vi "Get Device Channel Info.vi"(8 "error in":errorcluster, 10 "Channel Data in":T1 {"Device Chan Total" max=32 step=1; "Thermocouple"."Temperature Units" items=["Celcius", "Fahrenheit", "Kelvin", "Rankine", "Volts"]; "Thermocouple"."Thermocouple Type" items=["J", "K", "T", "E", "N", "B", "R", "S", "Raw Voltage"]}, 11 "Custom Device Ref in":T5 format="%.0x") -> (0 "error out":errorcluster, 2 "Channel Data out":T1 {"Device Chan Total" max=32 step=1; "Thermocouple"."Temperature Units" items=["Celcius", "Fahrenheit", "Kelvin", "Rankine", "Volts"]; "Thermocouple"."Thermocouple Type" items=["J", "K", "T", "E", "N", "B", "R", "S", "Raw Voltage"]}, 3 "Device Configuration Data":T4 {"Current Section Ref" format="%.0x"; "simTC Section Refs" format="%.0x"; "Voltage Section Ref" format="%.0x"; "Custom Device Ref" format="%.0x"})   [LabVIEW 2011, in "Simulated Thermocouple Custom Device.lvlib"]
uses:
  Simulated Thermocouple Custom Device.lvlib
  <vilib>/NI Veristand/Custom Device API/Custom Device Item Ref.ctl
  Device Config data.ctl
  New Channel Data.ctl
  TC Selector.ctl
  TC Unit Selector.ctl
  Device Settings.ctl
  TC Section Config Data.ctl
  <vilib>/NI Veristand/Custom Device API/Get Item Property (Variant).vi
  simTC Global GUIDs.vi
  <vilib>/NI Veristand/Custom Device Tools/Custom Device Utility Library/NI VeriStand - Search for All Items by GUID.vi
  <vilib>/NI Veristand/Custom Device Tools/Custom Device Utility Library/NI VeriStand - Search for Item by GUID.vi
  <vilib>/NI Veristand/Custom Device API/Get Item Property (String).vi
  <vilib>/NI Veristand/Custom Device Tools/Custom Device Utility Library/Custom Device Utility Library.lvlib
  <vilib>/NI Veristand/Custom Device API/Custom Device API.lvlib
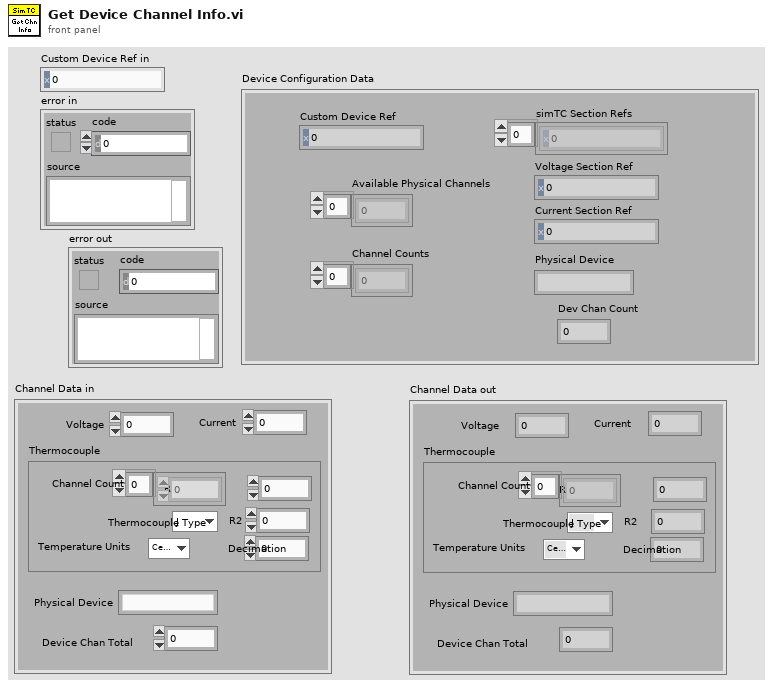
[diagram p1: front panel]
types:
  T1 = typedef "Simulated Thermocouple Custom Device.lvlib/New Channel Data.ctl" = cluster{"Voltage":u32, "Current":u32, "Thermocouple":cluster{"R1":dbl, "R2":dbl, "Decimation":u32, "Thermocouple Type":T2, "Temperature Units":T3, "Channel Count":u32[]}, "Physical Device":string, "Device Chan Total":u32}
  T2 = typedef "Simulated Thermocouple Custom Device.lvlib/TC Selector.ctl" = u16
  T3 = typedef "Simulated Thermocouple Custom Device.lvlib/TC Unit Selector.ctl" = u16
  T4 = typedef "Simulated Thermocouple Custom Device.lvlib/Device Config data.ctl" = cluster{"Custom Device Ref":T5, "Voltage Section Ref":T5, "simTC Section Refs":T5[], "Current Section Ref":T5, "Physical Device":string, "Available Physical Channels":i32[], "Channel Counts":u32[], "Dev Chan Count":u32}
  T5 = typedef "Custom Device API.lvlib/Custom Device Item Ref.ctl" = u64
  T6 = typedef "Simulated Thermocouple Custom Device.lvlib/Device Settings.ctl" = cluster{"High Side Resistance (Ohms)":dbl, "Low Side Resistance (Ohms)":dbl, "Temperature Units":T3, "Update Rate":dbl, "Physical Device Name":string, "Device Channel Count":u32}
  T7 = typedef "Simulated Thermocouple Custom Device.lvlib/TC Section Config Data.ctl" = cluster{"Temperature Units":T3, "Thermocouple Type":T2}
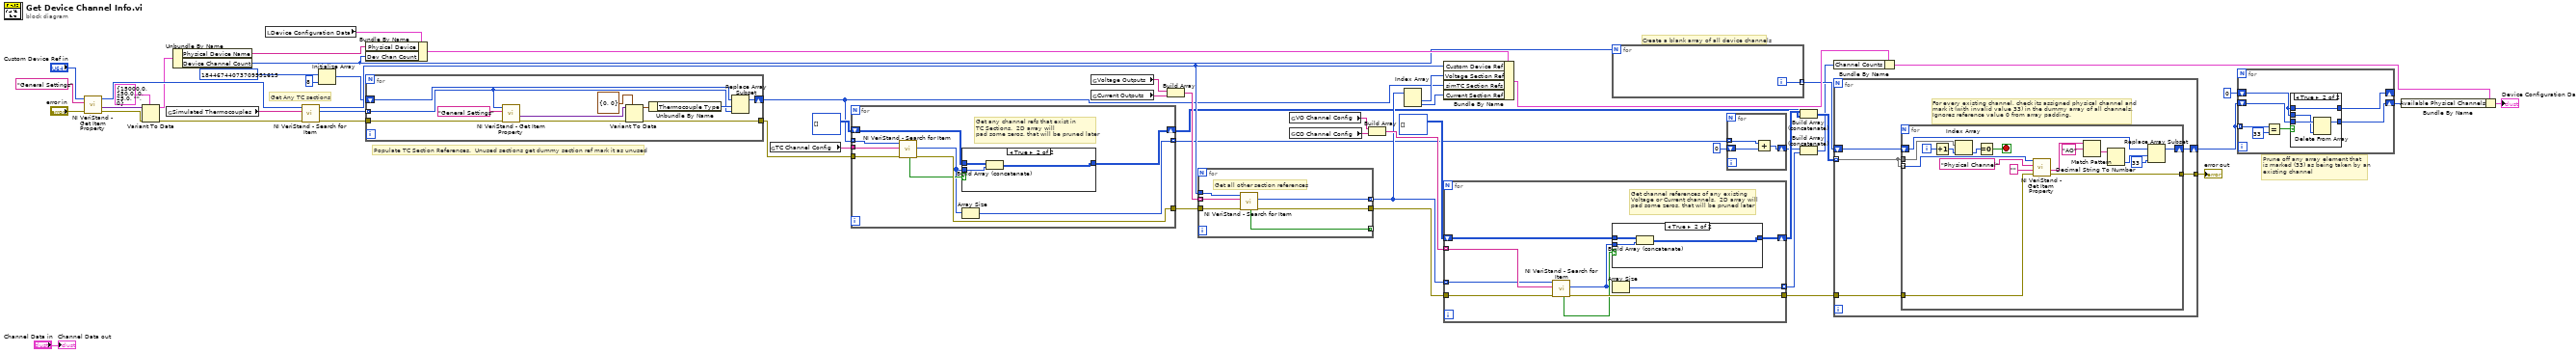
[diagram p0: block diagram]
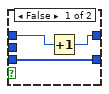
[diagram p3: hidden frame]
diagram:
  # "Populate TC Section References.  Unused sections get dummy section ref mark it as unused"
  # "Prune off any array element that\nis marked (33) as being taken by an\nexisting channel"
  # "Create a blank array of all device channels"
  # "Get Any TC sections"
  n1 = call-poly <vilib>:"NI VeriStand - Get Item Property.vi"("error in (no error)"="error in", "Property Name"="General Settings", "Item Ref in"="Custom Device Ref in") -> ("error out"=w3:errorcluster, "Value"=w2:variant, "Item Ref out"=w10:T5)  [unwired: 5 in, 1 out]
  n2 = Variant To Data(error in=w3, type=T6 {"High Side Resistance (Ohms)"=15000.0, "Low Side Resistance (Ohms)"=150.0, "Temperature Units"=0, "Update Rate"=25.0, "Physical Device Name"="", "Device Channel Count"=0} ("General Settings"), Variant=w2) -> (data=w9:T6, error out=w11:errorcluster)
  n3 = global read "simTC Global GUIDs.vi" "Simulated Thermocouples"() -> (w32:string)
  n4 = Unbundle By Name(w9) -> ("Physical Device Name"=w6:string, "Device Channel Count"=w8:u32)
  n5 = local read "Device Configuration Data"() -> (w37:T4)
  n6 = call-poly <vilib>:"NI VeriStand - Search for Item.vi"("error in"=w11, "Item GUID"=w32, "Section Ref in"=w10) -> ("error out"=w28:errorcluster, "Item Refs"=w4:T5[], "Section Ref out"=w31:T5)  [unwired: 5 in, 1 out]
  n7 = Initialize Array(T5 18446744073709551615 ("y"), 8 ("dimension size")) -> (w29:T5[])
  n8 = Bundle By Name(cluster=w37, "Physical Device"=w6, "Dev Chan Count"=w8) -> (w36:T4)
  n9 = for {
    tunnel: w4 -> [w59] mode=indexing
    shift-right: [w58] -> w7
    shift-left: w29 -> [w61]
    tunnel: w28 -> [w57]
    tunnel: [w56] -> w26
    n10 = call-poly <vilib>:"NI VeriStand - Get Item Property.vi"("error in (no error)"=w57, "Property Name"="General Settings", "Item Ref in"=w59) -> ("error out"=w63:errorcluster, "Value"=w64:variant)  [unwired: 5 in, 2 out]
    n11 = Variant To Data(error in=w63, type=T7 {"Temperature Units"=0, "Thermocouple Type"=0} ("TC Section Config Data"), Variant=w64) -> (data=w62:T7, error out=w56:errorcluster)
    n12 = Unbundle By Name(w62) -> ("Thermocouple Type"=w60:T2)
    n13 = Replace Array Subset(array=w61, new element=w59, index=w60) -> (w58:T5[])
  }
  n14 = global read "simTC Global GUIDs.vi" "TC Channel Config"() -> (w24:string)
  n15 = for {
    tunnel: w24 -> [w74]
    tunnel: w7 -> [w73] mode=indexing
    tunnel: w26 -> [w72]
    tunnel: [w71] -> w25
    tunnel: [w70] -> w16 mode=indexing
    shift-right: [w67] -> w20
    shift-left: i32[][] [] -> [w68]
    # "Get any channel refs that exist in\nTC Sections.  2D array will \npad some zeros, that will be pruned later"
    n16 = call-poly <vilib>:"NI VeriStand - Search for Item.vi"("error in"=w72, "Item GUID"=w74, "Section Ref in"=w73) -> ("error out"=w71:errorcluster, "Item Refs"=w66:T5[], "Found"=w69:bool)  [unwired: 5 in, 1 out]
    n17 = case shown="True" w69 {
      tunnel: w66 -> [_ w78]
      tunnel: w68 -> [w75 w77]
      tunnel: [w75 w76] -> w67
      frame False {
      }
      frame True {
        n18 = Build Array (concatenate)(w77, w78) -> (w76:T5[][])
      }
    }
    n19 = Array Size(array=w66) -> (size(s)=w70:i32)
  }
  n20 = global read "simTC Global GUIDs.vi" "Voltage Outputs"() -> (w54:string)
  n21 = global read "simTC Global GUIDs.vi" "Current Outputs"() -> (w53:string)
  n22 = Build Array(w54, w53) -> (w52:string[])
  n23 = for {
    tunnel: w31 -> [w84]
    tunnel: w52 -> [w83] mode=indexing
    tunnel: w25 -> [w82]
    tunnel: [w81] -> w27 mode=indexing
    tunnel: [w80] -> w51
    tunnel: [w79] -> _ mode=indexing
    # "Get all other section references"
    n24 = call-poly <vilib>:"NI VeriStand - Search for Item.vi"("error in"=w82, "Item GUID"=w83, "Section Ref in"=w84) -> ("error out"=w80:errorcluster, "Item Ref"=w81:T5, "Found"=w79:bool)  [unwired: 5 in, 1 out]
  }
  n25 = global read "simTC Global GUIDs.vi" "VO Channel Config"() -> (w47:string)
  n26 = global read "simTC Global GUIDs.vi" "CO Channel Config"() -> (w48:string)
  n27 = Build Array(w47, w48) -> (w46:string[])
  n28 = Index Array(array=w27) -> (element #1=w50:T5, element #2=w49:T5)  [unwired: 2 in]
  n29 = Bundle By Name(cluster=w36, "Custom Device Ref"=w31, "Voltage Section Ref"=w50, "simTC Section Refs"=w7, "Current Section Ref"=w49) -> (w45:T4)
  n30 = for {
    tunnel: w46 -> [w93] mode=indexing
    tunnel: w27 -> [w92] mode=indexing
    tunnel: w51 -> [w91]
    tunnel: [w90] -> w44
    tunnel: [w89] -> w18 mode=indexing
    shift-right: [w85] -> w22
    shift-left: i32[][] [] -> [w86]
    # "Get channel references of any existing\nVoltage or Current channels.  2D array will \npad some zeros, that will be pruned later"
    n31 = call-poly <vilib>:"NI VeriStand - Search for Item.vi"("error in"=w91, "Item GUID"=w93, "Section Ref in"=w92) -> ("error out"=w90:errorcluster, "Item Refs"=w87:T5[], "Found"=w88:bool)  [unwired: 5 in, 1 out]
    n32 = case shown="True" w88 {
      tunnel: w87 -> [_ w97]
      tunnel: w86 -> [w94 w96]
      tunnel: [w94 w95] -> w85
      frame False {
      }
      frame True {
        n33 = Build Array (concatenate)(w96, w97) -> (w95:T5[][])
      }
    }
    n34 = Array Size(array=w87) -> (size(s)=w89:i32)
  }
  n35 = for {
    N: w8 -> [_]
    tunnel: [w98] -> w35 mode=indexing
    i -> [w98]
  }
  n36 = for {
    tunnel: w16 -> [w101] mode=indexing
    shift-right: [w99] -> w14
    shift-left: 0 -> [w100]
    n37 = Add(x=w101, y=w100) -> (x+y=w99:i32)
  }
  n38 = Build Array (concatenate)(w22, w20) -> (w21:T5[][])
  n39 = Build Array (concatenate)(w14, w18) -> (w19:i32[])
  n40 = Bundle By Name(cluster=w45, "Channel Counts"=w19) -> (w40:T4)
  n41 = for {
    tunnel: w21 -> [w102] mode=indexing
    tunnel: w44 -> [w105]
    shift-right: [w104] -> w42
    shift-left: w35 -> [w106]
    tunnel: [w103] -> w41
    # "For every existing channel, check its assigned physical channel and \nmark it (with invalid value 33) in the dummy array of all channels.  \nIgnores reference value 0 from array padding."
    n42 = for {
      tunnel: w102 -> [w119] mode=indexing
      tunnel: w105 -> [w122]
      tunnel: [w120] -> w103
      shift-right: [w121] -> w104
      shift-left: w106 -> [w123]
      tunnel: w102 -> [w111]
      i -> [w109]
      stop <- w107 stop-if-true
      n43 = Increment(x=w109) -> (x+1=w110:i32)
      n44 = Index Array(array=w111, index=w110) -> (element=w108:T5)
      n45 = Equal To 0?(x=w108) -> (x = 0?=w107:bool)
      n46 = call-poly <vilib>:"NI VeriStand - Get Item Property.vi"("error in (no error)"=w122, "Default Value"="", "Property Name"="Physical Channel", "Item Ref in"=w119) -> ("error out"=w120:errorcluster, "Value"=w117:string)  [unwired: 4 in, 2 out]
      n47 = Match Pattern(string=w117, regular expression="AO") -> (after substring=w115:string)  [unwired: 1 in, 3 out]
      n48 = Decimal String To Number(string=w115) -> (number=w114:i32)  [unwired: 2 in, 1 out]
      n49 = Replace Array Subset(array=w123, new element=33 ("new element/subarray"), index=w114) -> (w121:i32[])
    }
  }
  "error out" <- w41
  n50 = for {
    shift-right: [w126] -> w39
    shift-left: w42 -> [w127]
    tunnel: w42 -> [w130] mode=indexing
    shift-right: [w125] -> _
    shift-left: 0 ("y") -> [w124]
    n51 = Equal?(x=w130, y=33) -> (x = y?=w128:bool)
    n52 = case shown="True" w128 {
      tunnel: w127 -> [w133 w137]
      tunnel: w124 -> [_ w136]
      tunnel: [w133 w135] -> w126
      tunnel: [w132 w134] -> w125
      tunnel: w124 -> [w131 w134]
      frame False {
        n53 = Increment(x=w131) -> (x+1=w132:i32)
      }
      frame True {
        n54 = Delete From Array(array=w137, index=w136) -> (array with subset deleted=w135:i32[])  [unwired: 1 in, 1 out]
      }
    }
  }
  n55 = Bundle By Name(cluster=w40, "Available Physical Channels"=w39) -> (→"Device Configuration Data":T4)
  "Channel Data out" <- "Channel Data in"
